vi "DefenderNormal.vi"(4 "IA State Input 2":T1={"our_robots"=[], "enemy_robots"=[], "balls"=[], "geometry"={"line_width"=0, "field_length"=0, "field_width"=0, "boundary_width"=0, "referee_width"=0, "goal_width"=0, "goal_depth"=0, "goal_wall_width"=0, "center_circle_radius"=0, "defense_radius"=0, "defense_stretch"=0, "free_kick_from_defense_dist"=0, "penalty_spot_from_field_line_dist"=0, "penalty_line_from_spot_dist"=0}, "IA Judge"={"stage"="", "command"="", "our_goalie_id"=0.0, "enemy_goalie_id"=0.0, "command enum"=enum."Halt", "Time"=enum."Azul"}, "Received Timestamp"=timestamp(0 s since 1904-01-01), "Events"={"Touch"=FALSE, "Ball out"=FALSE, "id touch"=0.0, "Ball out of \nVision"=FALSE, "Ball inside \nGoalie area"=FALSE, "Robot not responding"=FALSE, "Robots responding status"=[1.0, 1.0, 1.0, 1.0, 1.0, 1.0], "Enemy Ball \nPossession"=FALSE, "Pass State"=FALSE, "id end of pass"=0.0, "Kick"=FALSE, "Id Possession"=0.0}}, 5 "Stop?":bool, 6 "Defensores":u32[](array[numeric]), 7 "total":i32, 8 "Field defense":dbl[](array[numeric]), 9 "Field Size in":T6, 10 "balls":T5[](array[typedef]), 11 "Our Robot in":T2={"id"=0, "function"=enum."Attacker", "x"=0.0, "y"=0.0, "orientation"=0.0, "v_tangent"=0.0, "v_normal"=0.0, "v_ang"=0.0, "kick_x"=0.0, "kick_z"=0.0, "dribble"=FALSE, "Timestamp"=timestamp(0 s since 1904-01-01), "dest_x"=0.0, "dest_y"=0.0, "dest_orientation"=0.0, "estimatives"={"est_v_tangent"=0.0, "est_v_normal"=0.0, "est_vx"=0.0, "est_vy"=0.0}, "dest_x_kick"=0.0, "dest_y_kick"=0.0, "Gap Coord"=[], "States"=enum."GoToTangent"}) -> (2 "Robot out":T2={"id"=0, "function"=enum."Attacker", "x"=0.0, "y"=0.0, "orientation"=0.0, "v_tangent"=0.0, "v_normal"=0.0, "v_ang"=0.0, "kick_x"=0.0, "kick_z"=0.0, "dribble"=FALSE, "Timestamp"=timestamp(0 s since 1904-01-01), "dest_x"=0.0, "dest_y"=0.0, "dest_orientation"=0.0, "estimatives"={"est_v_tangent"=0.0, "est_v_normal"=0.0, "est_vx"=0.0, "est_vy"=0.0}, "dest_x_kick"=0.0, "dest_y_kick"=0.0, "Gap Coord"=[], "States"=enum."GoToTangent"})   [LabVIEW 2016]
uses:
  Core/AI Robot.ctl
  Functions Enum.ctl
  AttackerStates.ctl
  Core/AI Ball.ctl
  Core/Field Size.ctl
  Core/AI Input.ctl
  Core/AI Judge.ctl
  Command Enum.ctl
  Util/Events/Events.ctl
panel:
  in  "D max":dbl=1700.0
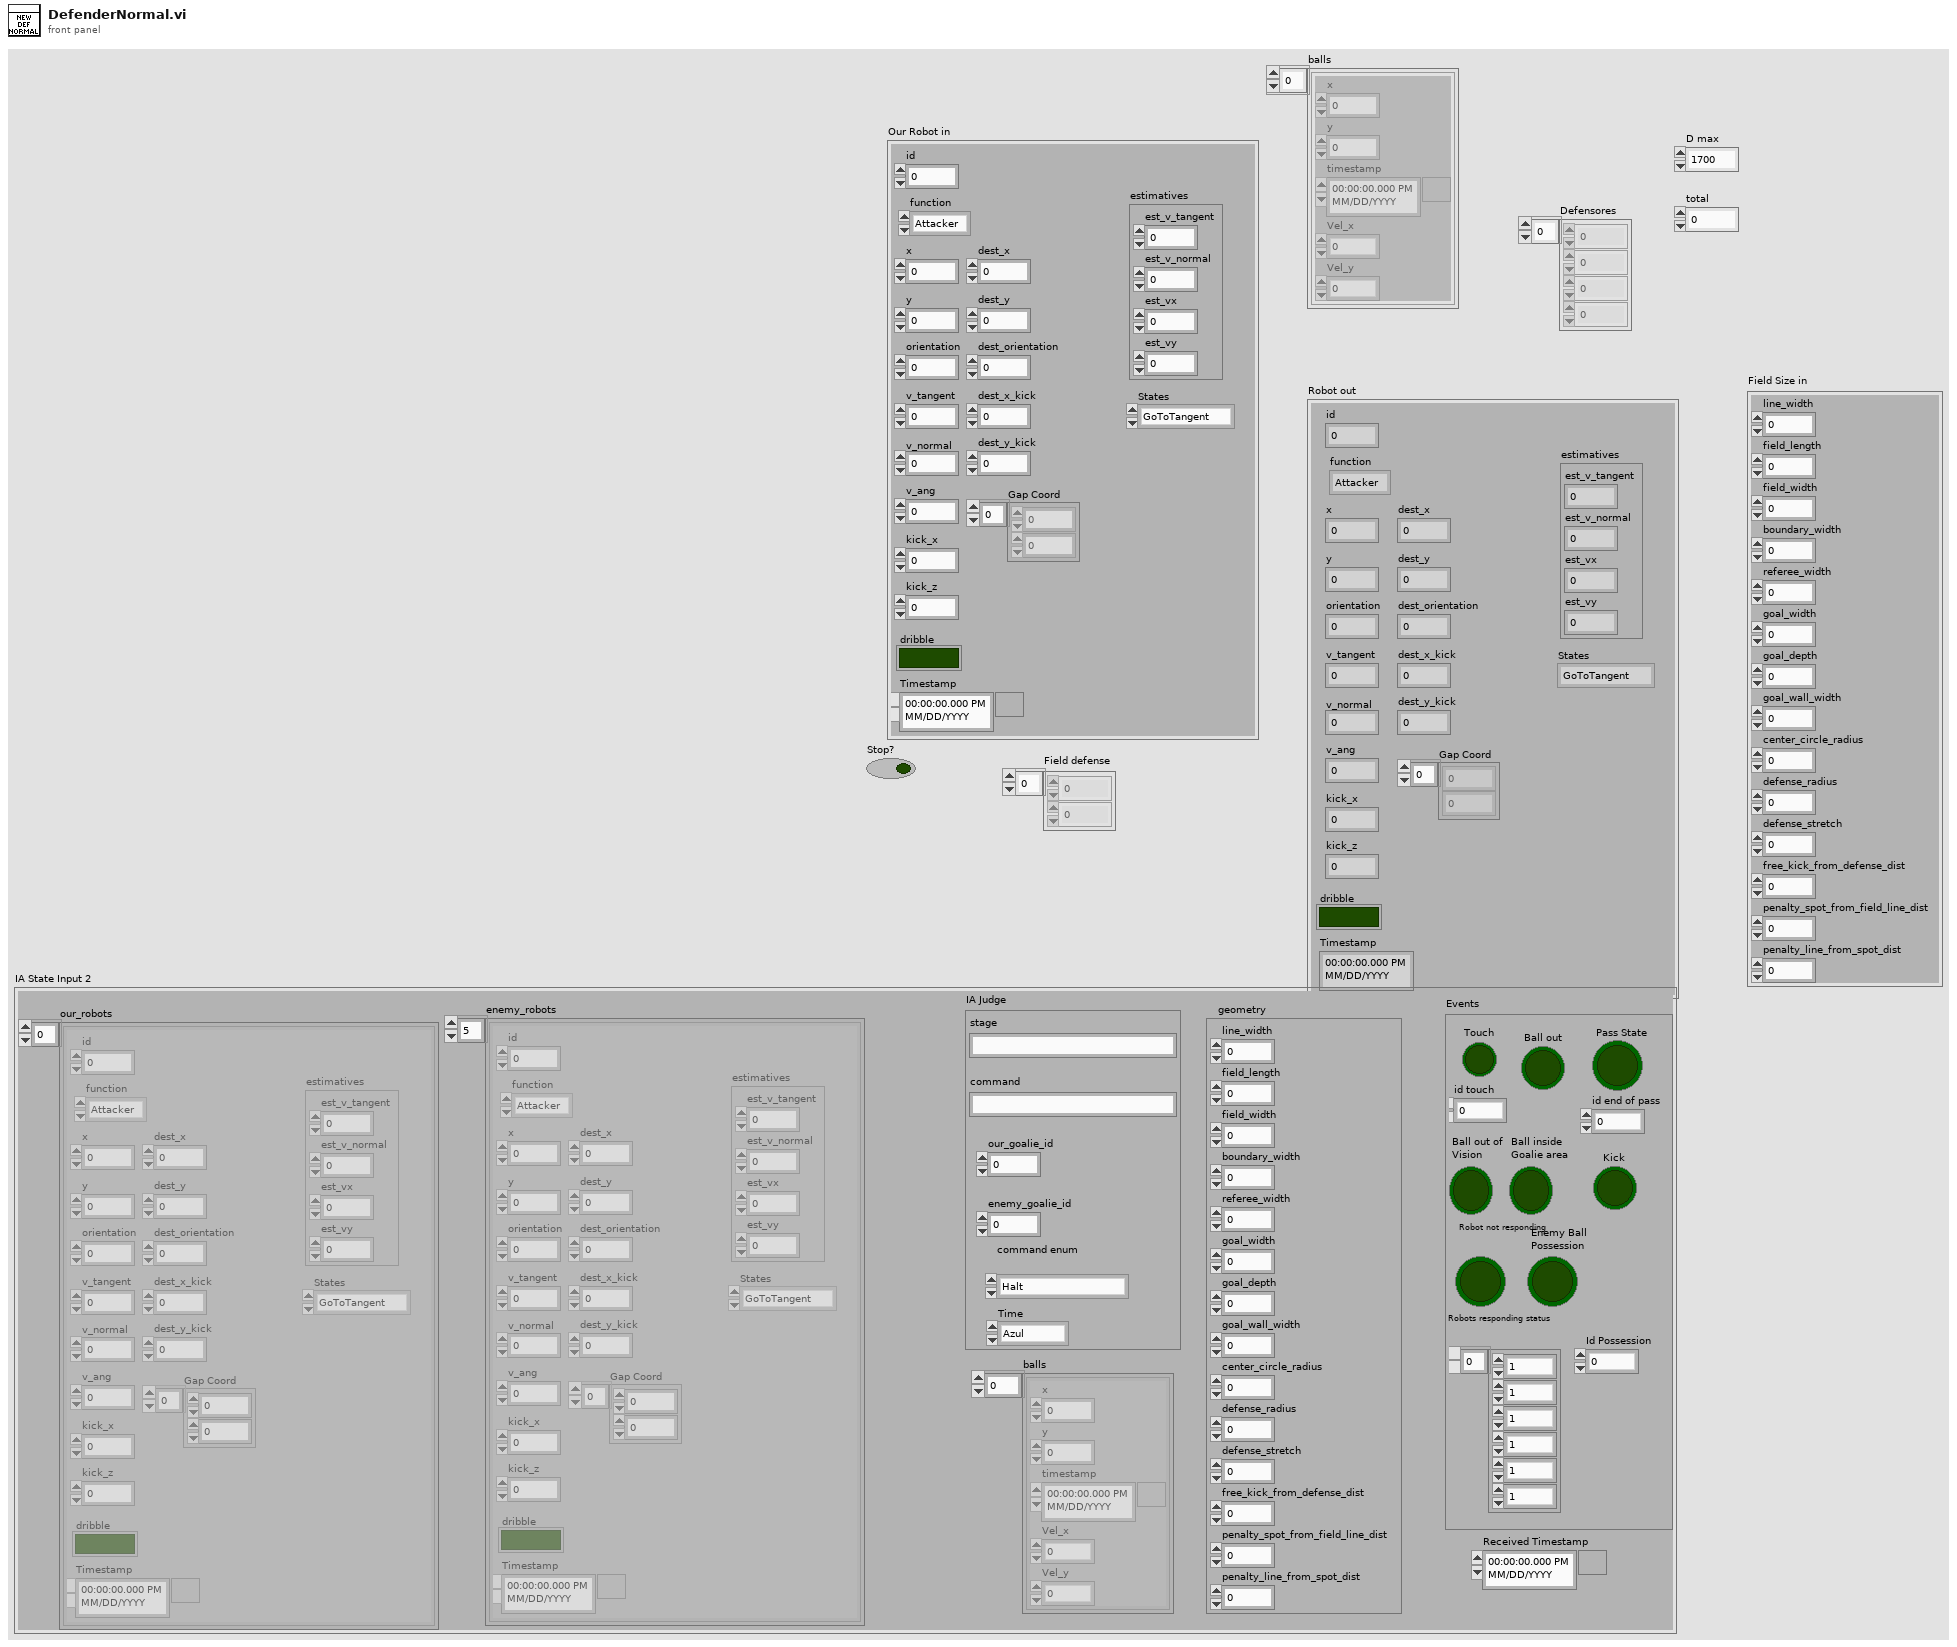
[diagram p1: front panel]
types:
  T1 = typedef "AI Input.ctl" = cluster{"our_robots":T2[], "enemy_robots":T2[], "balls":T5[], "geometry":T6, "IA Judge":T7, "Received Timestamp":timestamp, "Events":T9}
  T2 = typedef "AI Robot.ctl" = cluster{"id":u32, "function":T3, "x":dbl, "y":dbl, "orientation":dbl, "v_tangent":dbl, "v_normal":dbl, "v_ang":dbl, "kick_x":dbl, "kick_z":dbl, "dribble":bool, "Timestamp":timestamp, "dest_x":dbl, "dest_y":dbl, "dest_orientation":dbl, "estimatives":cluster{"est_v_tangent":dbl, "est_v_normal":dbl, "est_vx":dbl, "est_vy":dbl}, "dest_x_kick":dbl, "dest_y_kick":dbl, "Gap Coord":dbl[], "States":T4}
  T3 = typedef "Functions Enum.ctl" = enum16{"Attacker", "Goalie", "Defender", "Striker", "Goto 0", "Dummy", "Kicker", "ZigZag"}
  T4 = typedef "AttackerStates.ctl" = enum16{"Pass", "GoToTangent", "BallGetting", "GoToKick", ""}
  T5 = typedef "AI Ball.ctl" = cluster{"x":dbl, "y":dbl, "timestamp":timestamp, "Vel_x":dbl, "Vel_y":dbl}
  T6 = typedef "Field Size.ctl" = cluster{"line_width":u32, "field_length":u32, "field_width":u32, "boundary_width":u32, "referee_width":u32, "goal_width":u32, "goal_depth":u32, "goal_wall_width":u32, "center_circle_radius":u32, "defense_radius":u32, "defense_stretch":u32, "free_kick_from_defense_dist":u32, "penalty_spot_from_field_line_dist":u32, "penalty_line_from_spot_dist":u32}
  T7 = typedef "AI Judge.ctl" = cluster{"stage":string, "command":string, "our_goalie_id":dbl, "enemy_goalie_id":dbl, "command enum":T8, "Time":enum16{"Azul", "Amarelo"}}
  T8 = typedef "Command Enum.ctl" = enum16{"Halt", "Stop", "Force Start", "PKA Normal Start", "Prepare Kickoff Ally", "PKE Normal Start", "Prepare Kickoff Enemy", "Prepare Penalty Ally", "PPA Normal Start", "Prepare Penalty Enemy", "PPE Normal Start", "Direct Free Enemy", "Direct Free Ally", "Indirect Free Enemy", "Indirect Free Ally", "Timeout Enemy", "Timeout Ally", "Goal Enemy", "Goal Ally", "Ball Placement Enemy", "Ball Placement Ally", "Normal Half Time", "Extra Time Break", "Extra Half Time", "None"}
  T9 = typedef "Events.ctl" = cluster{"Touch":bool, "Ball out":bool, "id touch":dbl, "Ball out of \nVision":bool, "Ball inside \nGoalie area":bool, "Robot not responding":bool, "Robots responding status":dbl[], "Enemy Ball \nPossession":bool, "Pass State":bool, "id end of pass":dbl, "Kick":bool, "Id Possession":dbl}
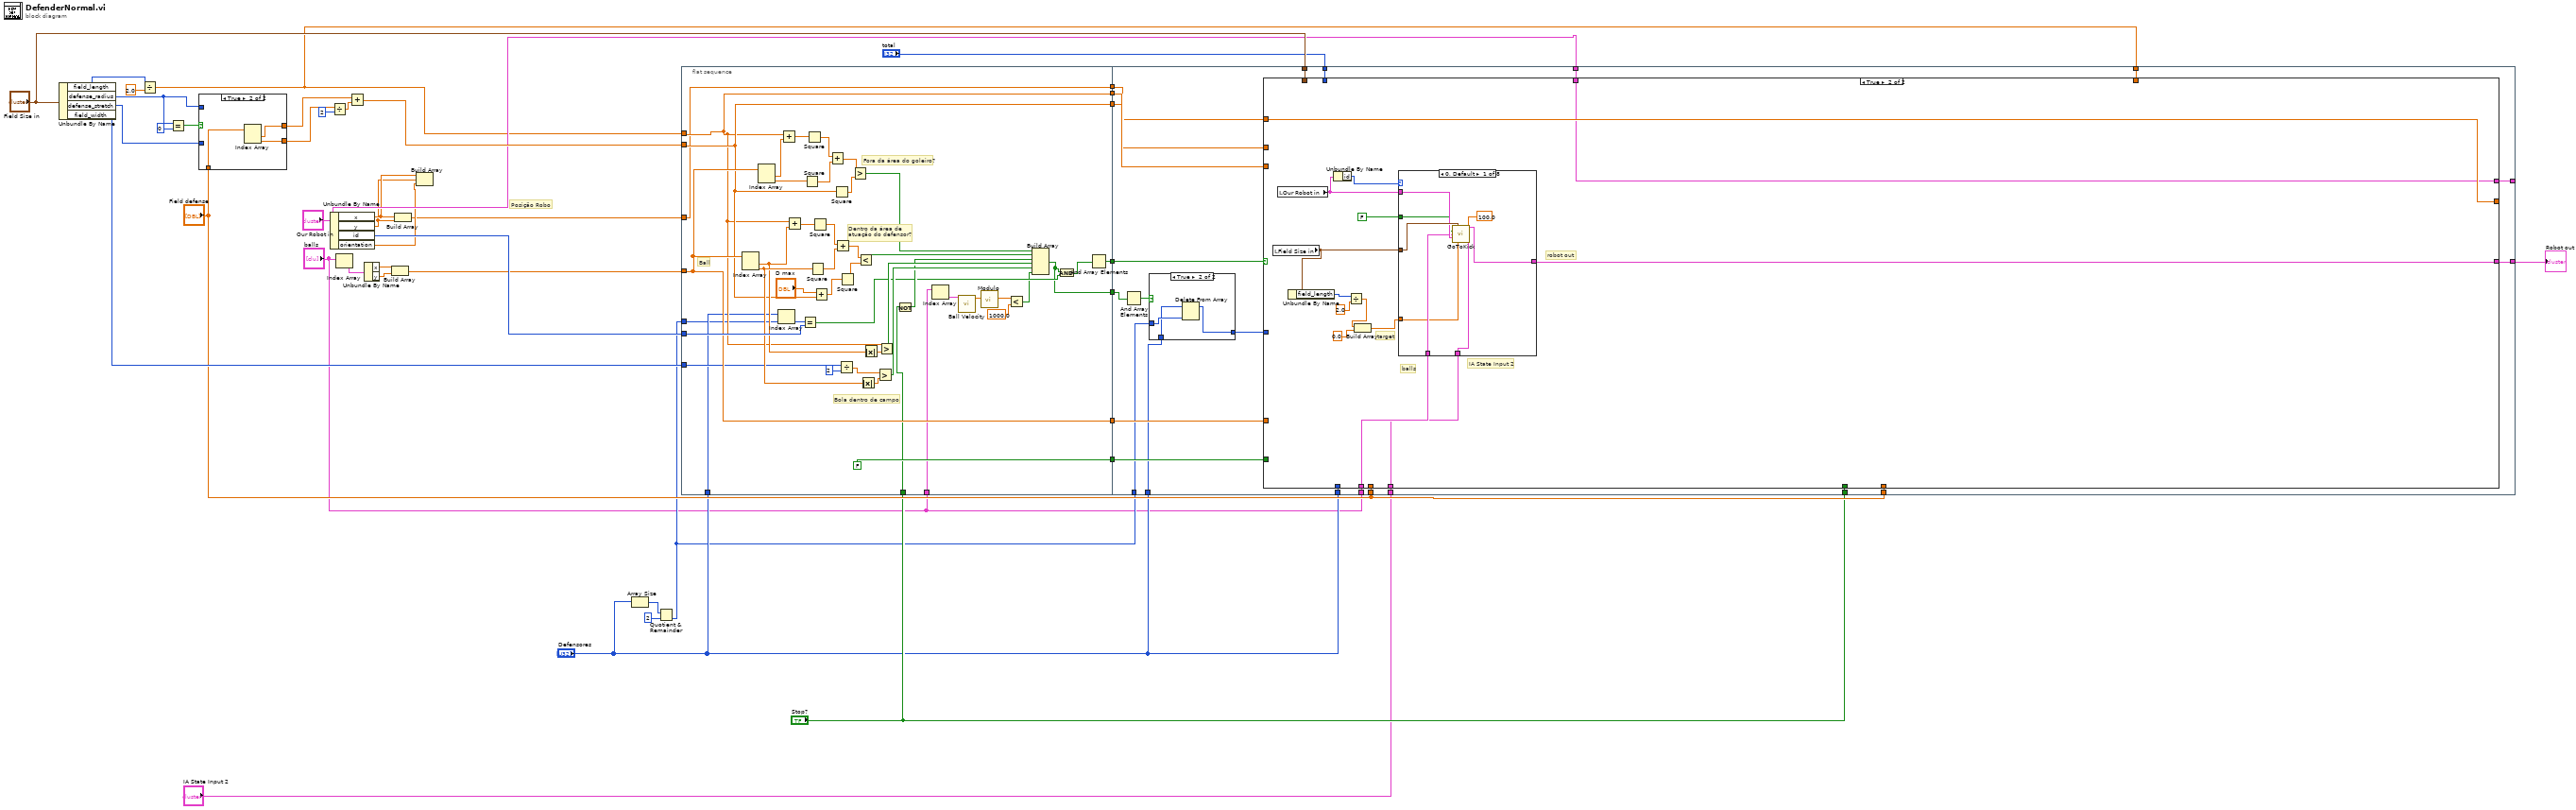
[diagram p0: block diagram]
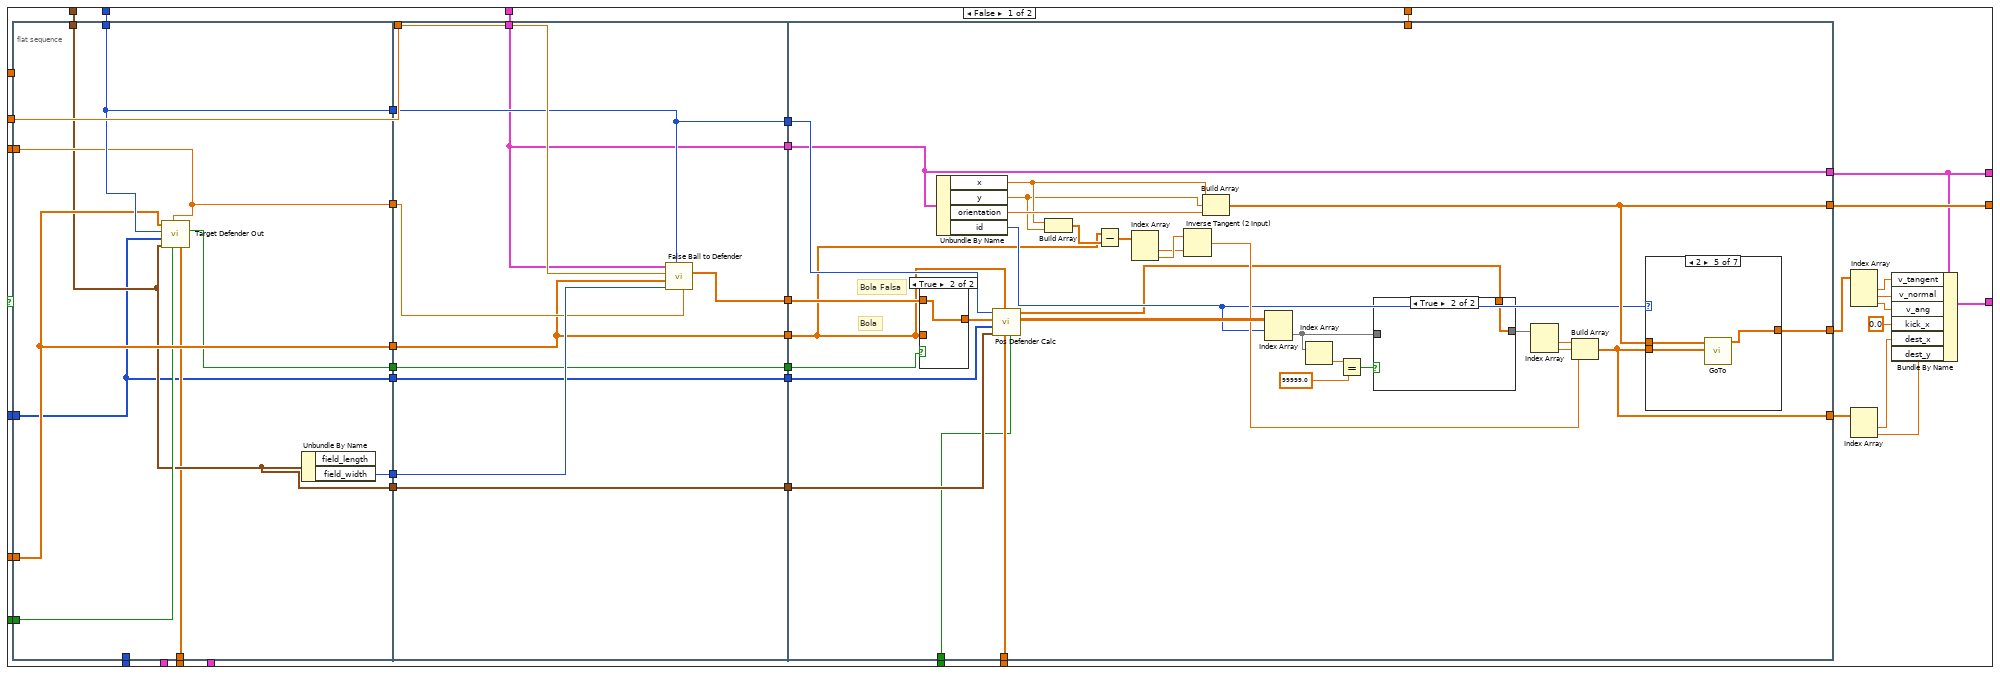
[diagram p4: hidden frame]
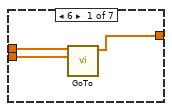
[diagram p6: hidden frame]
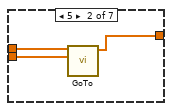
[diagram p7: hidden frame]
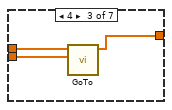
[diagram p8: hidden frame]
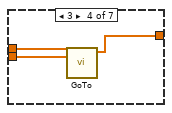
[diagram p9: hidden frame]
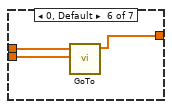
[diagram p10: hidden frame]
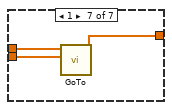
[diagram p11: hidden frame]
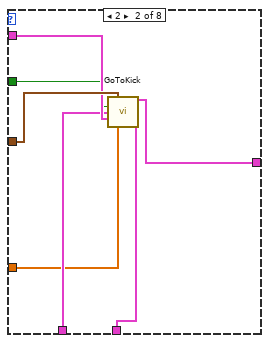
[diagram p13: hidden frame]
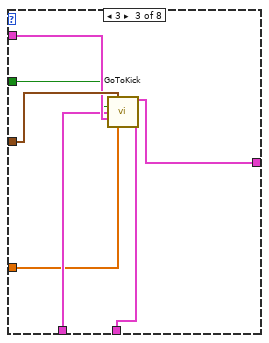
[diagram p14: hidden frame]
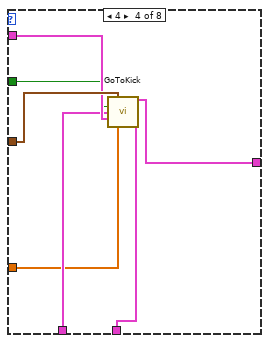
[diagram p15: hidden frame]
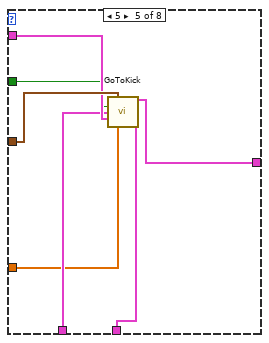
[diagram p16: hidden frame]
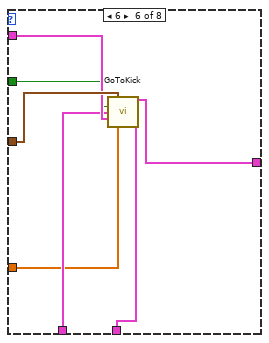
[diagram p17: hidden frame]
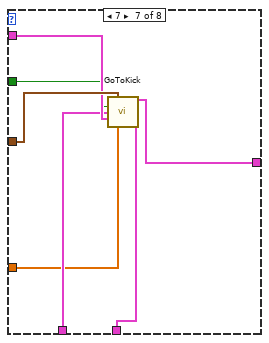
[diagram p18: hidden frame]
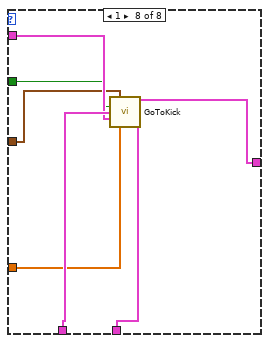
[diagram p19: hidden frame]
diagram:
  # "Posição Robo"
  n1 = Unbundle By Name("Field Size in") -> ("field_length"=w35:u32, "defense_radius"=w17:u32, "defense_stretch"=w16:u32, "field_width"=w32:u32)
  n2 = Divide(x=w35, y=2.0) -> (x/y=w7:dbl)
  n3 = Equal?(x=w17, y=u32 0) -> (x = y?=w15:bool)
  n4 = case shown="True" w15 {
    tunnel: [w43 w46] -> w14
    tunnel: w17 -> [w43 _]
    tunnel: w16 -> [w42 _]
    tunnel: [w42 w45] -> w13
    tunnel: "Field defense" -> [_ w44]
    frame False {
    }
    frame True {
      n5 = Index Array(array=w44) -> (element #1=w46:dbl, element #2=w45:dbl)  [unwired: 2 in]
    }
  }
  n6 = Unbundle By Name("Our Robot in") -> ("x"=w29:dbl, "y"=w28:dbl, "id"=w33:u32, "orientation"=w27:dbl)
  n7 = Divide(x=w13, y=u32 2) -> (x/y=w40:dbl)
  n8 = Index Array(array="balls") -> (element=w41:T5)  [unwired: 1 in]
  n9 = Add(x=w14, y=w40) -> (x+y=w34:dbl)
  n10 = Unbundle By Name(w41) -> ("x"=w38:dbl, "y"=w37:dbl)
  n11 = Build Array(w38, w37) -> (w8:dbl[])
  n12 = Build Array(w29, w28) -> (w10:dbl[])
  n13 = Build Array(w29, w28, w27) -> ()  [unwired: 1 out]
  n14 = Array Size(array="Defensores") -> (size(s)=w6:i32)
  n15 = Quotient & Remainder(x=w6, y=2) -> (floor(x/y)=w3:i32)  [unwired: 1 out]
  n16 = flat-sequence {
    tunnel: w34 -> [w63]
    tunnel: w7 -> [w62]
    tunnel: w8 -> [w79]
    tunnel: w10 -> [w61]
    tunnel: [w79] -> w26
    tunnel: [w84] -> w25
    tunnel: w33 -> [w83]
    tunnel: w32 -> [w70]
    tunnel: [FALSE ("Target Fora")] -> w24
    tunnel: [w62] -> w23
    tunnel: [w63] -> w22
    tunnel: [w61] -> w21
    tunnel: "Defensores" -> [w59]
    tunnel: "Stop?" -> [w58]
    tunnel: w3 -> [w57]
    tunnel: [w53] -> w2
    tunnel: "balls" -> [w51]
    tunnel: "total" -> [w115]
    tunnel: [w114] -> w19
    tunnel: w26 -> [w113]
    tunnel: w25 -> [w112]
    tunnel: w24 -> [w111]
    tunnel: w23 -> [w109]
    tunnel: "Field Size in" -> [w110]
    tunnel: "Our Robot in" -> [w108]
    tunnel: w22 -> [w107]
    tunnel: [w106] -> _
    tunnel: w21 -> [w105]
    tunnel: "Field defense" -> [w104]
    tunnel: "Field defense" -> [w103]
    tunnel: "Defensores" -> [w102]
    tunnel: "IA State Input 2" -> [w101]
    tunnel: "balls" -> [w100]
    tunnel: "Stop?" -> [w99]
    tunnel: w7 -> [w98]
    tunnel: "Defensores" -> [w96]
    tunnel: w3 -> [w97]
    tunnel: w2 -> [w95]
    frame #0 {
      # "Bola dentro de campo"
      # "Dentro da área de \natuação do defensor?"
      # "Fora da área do goleiro?"
      # "Ball"
      n17 = Index Array(array=w79) -> (element #1=w67:dbl, element #2=w71:dbl)  [unwired: 2 in]
      n18 = Index Array(array=w79) -> (element #1=w85:dbl, element #2=w87:dbl)  [unwired: 2 in]
      n19 = Index Array(array=w59, index=w57) -> (element=w60:u32)
      n20 = Add(x=w62, y=w85) -> (x+y=w86:dbl)
      n21 = Add(x=w62, y=w67) -> (x+y=w80:dbl)
      n22 = Equal?(x=w60, y=w83) -> (x = y?=w55:bool)
      n23 = Square(x=w87) -> (x^2=w89:dbl)
      n24 = Square(x=w86) -> (x^2=w88:dbl)
      n25 = Square(x=w71) -> (x^2=w82:dbl)
      n26 = Square(x=w80) -> (x^2=w81:dbl)
      n27 = Add(x="D max", y=w63) -> (x+y=w65:dbl)
      n28 = Add(x=w88, y=w89) -> (x+y=w90:dbl)
      n29 = Square(x=w63) -> (x^2=w91:dbl)
      n30 = Add(x=w81, y=w82) -> (x+y=w76:dbl)
      n31 = Divide(x=w70, y=u32 2) -> (x/y=w73:dbl)
      n32 = Square(x=w65) -> (x^2=w78:dbl)
      n33 = Greater?(x=w90, y=w91) -> (0:w92:bool)
      n34 = Less?(x=w76, y=w78) -> (x < y?=w77:bool)
      n35 = Absolute Value(x=w71) -> (abs(x)=w72:dbl)
      n36 = Absolute Value(x=w67) -> (abs(x)=w75:dbl)
      n37 = Greater?(x=w73, y=w72) -> (0:w68:bool)
      n38 = Greater?(x=w62, y=w75) -> (0:w74:bool)
      n39 = Not(x=w58) -> (.not. x?=w56:bool)
      n40 = Index Array(array=w51) -> (element=w52:T5)  [unwired: 1 in]
      n41 = call "Ball Velocity.vi"("Ball"=w52) -> ("Velocity"=w49:dbl[])  [unwired: 10 in]
      n42 = call "Modulo.vi"("2D vector"=w49) -> ("Modulo"=w48:dbl)  [unwired: 10 in]
      n43 = Less?(x=w48, y=1000.0) -> (x < y?=w50:bool)
      n44 = Build Array(w92, w77, w56, w74, w68, w50) -> (w53:bool[])
      n45 = And(x=w53, y=w55) -> (x .and. y?=w54:bool[])
      n46 = And Array Elements(Boolean array=w54) -> (logical AND=w84:bool)
    }
    frame #1 {
      n47 = And Array Elements(Boolean array=w95) -> (logical AND=w94:bool)
      n48 = case shown="True" w94 {
        tunnel: w97 -> [_ w119]
        tunnel: w96 -> [w116 w118]
        tunnel: [w116 w117] -> w93
        frame False {
        }
        frame True {
          n49 = Delete From Array(array=w118, index=w119) -> (array with subset deleted=w117:u32[])  [unwired: 1 in, 1 out]
        }
      }
      n50 = case shown="True" w112 {
        tunnel: w115 -> [w156 _]
        tunnel: [w151 w242] -> w114
        tunnel: w113 -> [w150 _]
        tunnel: w111 -> [w148 _]
        tunnel: w109 -> [w147 _]
        tunnel: w110 -> [w146 _]
        tunnel: w108 -> [w145 w245]
        tunnel: w107 -> [w144 _]
        tunnel: [w130 w246] -> _
        tunnel: [w129 w245] -> w106
        tunnel: w105 -> [_ w246]
        tunnel: w104 -> [w128 _]
        tunnel: w103 -> [w127 _]
        tunnel: w102 -> [w126 _]
        tunnel: w101 -> [_ w243]
        tunnel: w100 -> [_ w244]
        tunnel: w99 -> [w125 _]
        tunnel: w98 -> [w124 _]
        tunnel: w93 -> [w120 _]
        frame False {
          n51 = flat-sequence {
            tunnel: w156 -> [w165]
            tunnel: [w166] -> w157
            tunnel: w150 -> [w164]
            tunnel: [w165] -> w149
            tunnel: w148 -> [w162]
            tunnel: w147 -> [w163]
            tunnel: w146 -> [w160]
            tunnel: [w164] -> w143
            tunnel: [w163] -> w142
            tunnel: [w161] -> w138
            tunnel: [w158] -> w135
            tunnel: [w160] -> w133
            tunnel: w127 -> [w159]
            tunnel: w126 -> [_]
            tunnel: w120 -> [w158]
            tunnel: w157 -> [w176]
            tunnel: w149 -> [w170]
            tunnel: w145 -> [w167]
            tunnel: w144 -> [w175]
            tunnel: w143 -> [w172]
            tunnel: w142 -> [w174]
            tunnel: [w173] -> w141
            tunnel: [w172] -> w140
            tunnel: [w171] -> w139
            tunnel: w138 -> [w171]
            tunnel: [w170] -> w137
            tunnel: [w169] -> w136
            tunnel: w135 -> [w169]
            tunnel: [w168] -> w134
            tunnel: w133 -> [w168]
            tunnel: [w167] -> w132
            tunnel: [w200] -> w131
            tunnel: [w195] -> w129
            tunnel: w141 -> [w199]
            tunnel: w140 -> [w184]
            tunnel: w139 -> [w198]
            tunnel: w137 -> [w197]
            tunnel: w136 -> [w196]
            tunnel: w134 -> [w194]
            tunnel: w132 -> [w195]
            tunnel: [w189] -> w130
            tunnel: w128 -> [w186]
            tunnel: w125 -> [w185]
            tunnel: w124 -> [_]
            tunnel: [w178] -> w123
            frame #0 {
              n52 = call "Target Defender Out.vi"("Field defense"=w159, "Target Fora in"=w162, "Campo/2"=w163, "Field Size in"=w160, "Defensores"=w158, "total"=w165, "Ball"=w164) -> ("Target Fora out"=w161:bool)  [unwired: 4 in]
              n53 = Unbundle By Name(w160) -> ("field_width"=w166:u32)  [unwired: 1 out]
            }
            frame #1 {
              n54 = call "False Ball to Defender.vi"("Campo/2"=w174, "field_width"=w176, "total"=w170, "Bola"=w172, "raio da área \ndo goleiro"=w175, "Our Robot in"=w167) -> ("Bola Falsa"=w173:dbl[])  [unwired: 5 in]
            }
            frame #2 {
              # "Bola"
              # "Bola Falsa"
              n55 = case shown="True" w198 {
                tunnel: [w231 w232] -> w207
                tunnel: w199 -> [_ w232]
                tunnel: w184 -> [w231 _]
                frame False {
                }
                frame True {
                }
              }
              n56 = Unbundle By Name(w195) -> ("x"=w205:dbl, "y"=w204:dbl, "orientation"=w206:dbl, "id"=w187:u32)
              n57 = call "Pos Defender Calc.vi"("Stop?"=w185, "Field defense"=w186, "Real Ball"=w184, "Field Size in"=w194, "Defensores"=w196, "Ball"=w207, "total"=w197) -> ("Posição dos Defensores"=w192:dbl[][], "Central Position"=w177:dbl[])  [unwired: 3 in]
              n58 = Build Array(w205, w204) -> (w193:dbl[])
              n59 = Subtract(x=w184, y=w193) -> (x-y=w203:dbl[])
              n60 = Index Array(array=w203) -> (element #1=w201:dbl, element #2=w202:dbl)  [unwired: 2 in]
              n61 = Inverse Tangent (2 Input)(1:w201, 2:w202) -> (0:w188:dbl)
              n62 = Build Array(w205, w204, w206) -> (w189:dbl[])
              n63 = Index Array(array=w192, index (row)=w187) -> (element=w182:dbl[])  [unwired: 1 in]
              n64 = Index Array(array=w182) -> (element=w181:dbl)  [unwired: 1 in]
              n65 = Equal?(x=w181, y=99999.0) -> (x = y?=w180:bool)
              n66 = case shown="True" w180 {
                tunnel: [w208 w209] -> w183
                tunnel: w182 -> [w208 _]
                tunnel: w177 -> [_ w209]
                frame False {
                }
                frame True {
                }
              }
              n67 = Index Array(array=w183) -> (element #1=w191:dbl, element #2=w190:dbl)  [unwired: 2 in]
              n68 = Build Array(w191, w190, w188) -> (w178:dbl[])
              n69 = case shown="2" w187 {
                tunnel: [w210 w213 w216 w219 w222 w225 w230] -> w200
                tunnel: w178 -> [w211 w215 w217 w220 w223 w226 w229]
                tunnel: w189 -> [w212 w214 w218 w221 w224 w227 w228]
                frame 6 {
                  n70 = call "GoTo.vi"("Target"=w211, "Position"=w212) -> ("Output\nVelocity"=w210:dbl[])  [unwired: 8 in, 1 out]
                }
                frame 5 {
                  n71 = call "GoTo.vi"("Target"=w215, "Position"=w214) -> ("Output\nVelocity"=w213:dbl[])  [unwired: 8 in, 1 out]
                }
                frame 4 {
                  n72 = call "GoTo.vi"("Target"=w217, "Position"=w218) -> ("Output\nVelocity"=w216:dbl[])  [unwired: 8 in, 1 out]
                }
                frame 3 {
                  n73 = call "GoTo.vi"("Target"=w220, "Position"=w221) -> ("Output\nVelocity"=w219:dbl[])  [unwired: 8 in, 1 out]
                }
                frame 2 {
                  n74 = call "GoTo.vi"("Target"=w223, "Position"=w224) -> ("Output\nVelocity"=w222:dbl[])  [unwired: 8 in, 1 out]
                }
                frame 0, Default {
                  n75 = call "GoTo.vi"("Target"=w226, "Position"=w227) -> ("Output\nVelocity"=w225:dbl[])  [unwired: 8 in, 1 out]
                }
                frame 1 {
                  n76 = call "GoTo.vi"("Target"=w229, "Position"=w228) -> ("Output\nVelocity"=w230:dbl[])  [unwired: 8 in, 1 out]
                }
              }
            }
          }
          n77 = Index Array(array=w131) -> (element #1=w154:dbl, element #2=w153:dbl, element #3=w152:dbl)  [unwired: 3 in]
          n78 = Index Array(array=w123) -> (element #1=w122:dbl, element #2=w121:dbl)  [unwired: 2 in]
          n79 = Bundle By Name(cluster=w129, "v_tangent"=w154, "v_normal"=w153, "v_ang"=w152, "kick_x"=0.0, "dest_x"=w122, "dest_y"=w121) -> (w151:T2)
        }
        frame True {
          # "target"
          # "robot out"
          # "IA State Input 2"
          # "balls"
          n80 = local read "Field Size in"() -> (w237:T6)
          n81 = local read "Our Robot in"() -> (w241:T2)
          n82 = Unbundle By Name(w237) -> ("field_length"=w236:u32)
          n83 = Unbundle By Name(w241) -> ("id"=w240:u32)
          n84 = Divide(x=w236, y=2.0) -> (x/y=w234:dbl)
          n85 = Build Array(w234, 0.0) -> (w239:dbl[])
          n86 = case shown="0, Default" w240 {
            tunnel: w241 -> [w253 w260 w267 w274 w281 w288 w295 w300]
            tunnel: w237 -> [w254 w261 w268 w275 w282 w289 w296 w298]
            tunnel: w244 -> [w252 w259 w266 w273 w280 w287 w294 w303]
            tunnel: w243 -> [w251 w258 w265 w272 w279 w286 w293 w301]
            tunnel: [w250 w257 w264 w271 w278 w285 w292 w299] -> w242
            tunnel: w239 -> [w249 w256 w263 w270 w277 w284 w291 w302]
            tunnel: FALSE -> [w248 w255 w262 w269 w276 w283 w290 w297]
            frame 0, Default {
              n87 = call "GoToKick.vi"("Field Size in"=w254, "goleiro?"=w248, "balls"=w252, "Robot in in"=w253, "Kick Force"=100.0, "Target"=w249, "IA State Input in"=w251) -> ("Robot out"=w250:T2)  [unwired: 6 in, 2 out]
            }
            frame 2 {
              n88 = call "GoToKick.vi"("Field Size in"=w261, "goleiro?"=w255, "balls"=w259, "Robot in in"=w260, "Target"=w256, "IA State Input in"=w258) -> ("Robot out"=w257:T2)  [unwired: 7 in, 2 out]
            }
            frame 3 {
              n89 = call "GoToKick.vi"("Field Size in"=w268, "goleiro?"=w262, "balls"=w266, "Robot in in"=w267, "Target"=w263, "IA State Input in"=w265) -> ("Robot out"=w264:T2)  [unwired: 7 in, 2 out]
            }
            frame 4 {
              n90 = call "GoToKick.vi"("Field Size in"=w275, "goleiro?"=w269, "balls"=w273, "Robot in in"=w274, "Target"=w270, "IA State Input in"=w272) -> ("Robot out"=w271:T2)  [unwired: 7 in, 2 out]
            }
            frame 5 {
              n91 = call "GoToKick.vi"("Field Size in"=w282, "goleiro?"=w276, "balls"=w280, "Robot in in"=w281, "Target"=w277, "IA State Input in"=w279) -> ("Robot out"=w278:T2)  [unwired: 7 in, 2 out]
            }
            frame 6 {
              n92 = call "GoToKick.vi"("Field Size in"=w289, "goleiro?"=w283, "balls"=w287, "Robot in in"=w288, "Target"=w284, "IA State Input in"=w286) -> ("Robot out"=w285:T2)  [unwired: 7 in, 2 out]
            }
            frame 7 {
              n93 = call "GoToKick.vi"("Field Size in"=w296, "goleiro?"=w290, "balls"=w294, "Robot in in"=w295, "Target"=w291, "IA State Input in"=w293) -> ("Robot out"=w292:T2)  [unwired: 7 in, 2 out]
            }
            frame 1 {
              n94 = call "GoToKick.vi"("Field Size in"=w298, "goleiro?"=w297, "balls"=w303, "Robot in in"=w300, "Target"=w302, "IA State Input in"=w301) -> ("Robot out"=w299:T2)  [unwired: 7 in, 2 out]
            }
          }
        }
      }
    }
  }
  "Robot out" <- w19
